vi "Init_Test.vi"(8 "error in (no error)":errorcluster caption="entrée d'erreur (pas d'erreur)", 11 "Get_Voltage en entrée":refnum<class "Disable_Power_Supply.lvclass">) -> (0 "error out":errorcluster caption="sortie d'erreur", 3 "Get_Voltage en sortie":refnum<class "Disable_Power_Supply.lvclass">)   [LabVIEW 2020, in "Library Test.lvlib" / "Disable_Power_Supply.lvclass"]
uses:
  Disable_Power_Supply.lvclass
  C:/Users/ngarcin/OneDrive - Altyor/Standard TB/Class/Test/Test (Default)/Test (Default).lvclass
  Commun VI/TypeDef/Commande Test/Commande Value Type.ctl
  Commun VI/TypeDef/Commande Test/Commande Type Test.ctl
  Commun VI/TypeDef/Command Power_Supply/Data_Write_Power_Supply.ctl
  JSON API/Variant JSON/Variant to JSON.vi
  JSON API/JSON Value/Get Item by name array.vi
  Test_Wtih_Instr/Test_With_Inst.lvclass
  Instrument/Instrument (Default)/Class Instrument (Default).lvclass
  JSON API/JSON Value/JSON Value.lvclass
  Disable_Power_Supply.lvclass/Disable_Power_Supply.ctl
  Commun VI/Library Commun.lvlib
  JSON API/Get Polymorphic/JSON GetSet.lvlib
  JSON API/Variant JSON/Variant JSON.lvlib
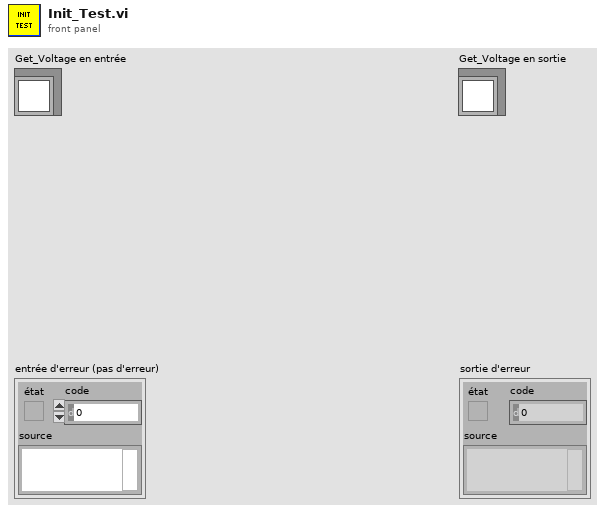
[diagram p1: front panel]
types:
  T1 = typedef "Library Commun.lvlib/Commande Type Test.ctl" = enum16{"Function", "Test", "Calculation"}
  T2 = typedef "Library Commun.lvlib/Commande Value Type.ctl" = enum16{"None", "String", "Number", "Timestamp", "Boolean", "Array"}
  T3 = typedef "Library Commun.lvlib/Data_Write_Power_Supply.ctl" = enum16{"Enable Channel", "Disable Channel"}
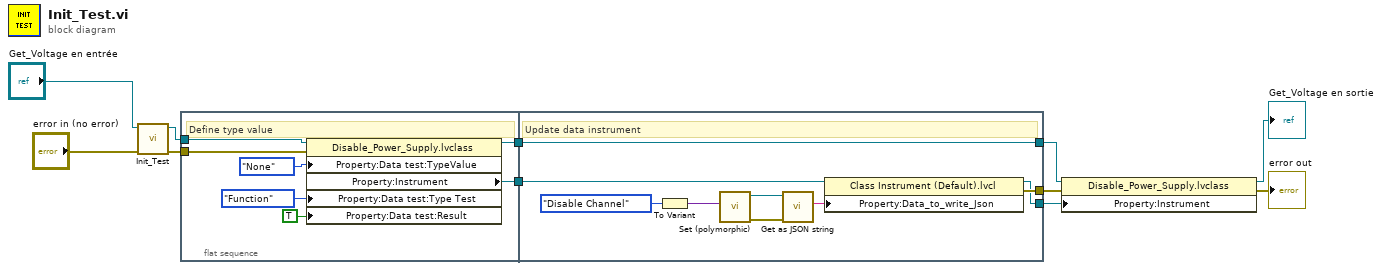
[diagram p0: block diagram]
diagram:
  n1 = call-parent "Init_Test.vi"("error in (no error)"="error in (no error)", "Test_With_Inst en entrée"="Get_Voltage en entrée") -> ("error out"=w8:errorcluster, "Test_With_Inst en sortie"=w9:refnum<class "Disable_Power_Supply.lvclass">)  [unwired: 8 in]
  n2 = flat-sequence {
    tunnel: w9 -> [w18]
    tunnel: w8 -> [w17]
    tunnel: [w15] -> w7
    tunnel: [w14] -> w6
    tunnel: [w27] -> w3
    tunnel: [w26] -> w4
    tunnel: w7 -> [w25]
    tunnel: [w25] -> w5
    tunnel: w6 -> [w20]
    frame #0 {
      # "Define type value"
      n3 = property class="Disable_Power_Supply.lvclass"(reference=w18, error in=w17, "Property:Data test:TypeValue"=Commande_Value_Type."None" ("TypeValue"), "Property:Data test:Type Test"=Commande_Type_Test."Function" ("Type Test"), "Property:Data test:Result"=TRUE ("Result")) -> (reference out=w15:refnum<class "Disable_Power_Supply.lvclass">, "Property:Instrument"=w14:refnum<class "Class Instrument (Default).lvclass">)  [unwired: 1 out]
    }
    frame #1 {
      # "Update data instrument"
      n4 = To Variant(anything=Data_Write_Power_Supply."Disable Channel" ("Function")) -> (Variant=w24:variant)
      n5 = call-poly "Set (polymorphic).vi"("Variant"=w24) -> ("error out"=w22:errorcluster, "JSON Value out"=w23:refnum<class "JSON Value.lvclass">)  [unwired: 9 in]
      n6 = call "Get as JSON string.vi"("error in (no error)"=w22, "JSON Value in"=w23) -> ("<JSON>"=w21:string)  [unwired: 8 in, 1 out]
      n7 = property class="Class Instrument (Default).lvcl"(reference=w20, "Property:Data_to_write_Json"=w21) -> (reference out=w26:refnum<class "Class Instrument (Default).lvclass">, error out=w27:errorcluster)  [unwired: 1 in]
    }
  }
  n8 = property class="Disable_Power_Supply.lvclass"(reference=w5, error in=w3, "Property:Instrument"=w4) -> (reference out=→"Get_Voltage en sortie":refnum<class "Disable_Power_Supply.lvclass">, error out=→"error out":errorcluster)
